vi "Pockels-Determine number of insertions for ref frame AO seq.vi"(7 "Prevent small final chunks (T)":bool, 9 "Nominal chunk length (points)":i32, 11 "Number of points in the original pockels modulation sequence":i32) -> (2 "Number of insertions":i32, 3 "Size of last chunk as % of nominal chunk size":dbl(slide) scale=0.0..100.0)   [LabVIEW 2020]
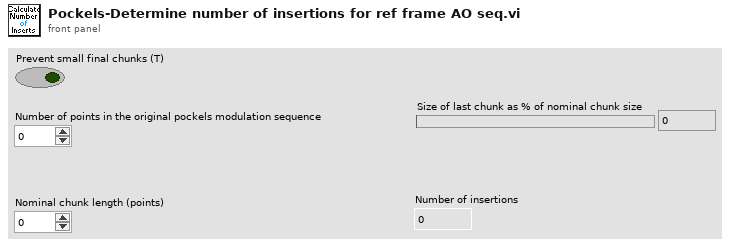
[diagram p1: front panel]
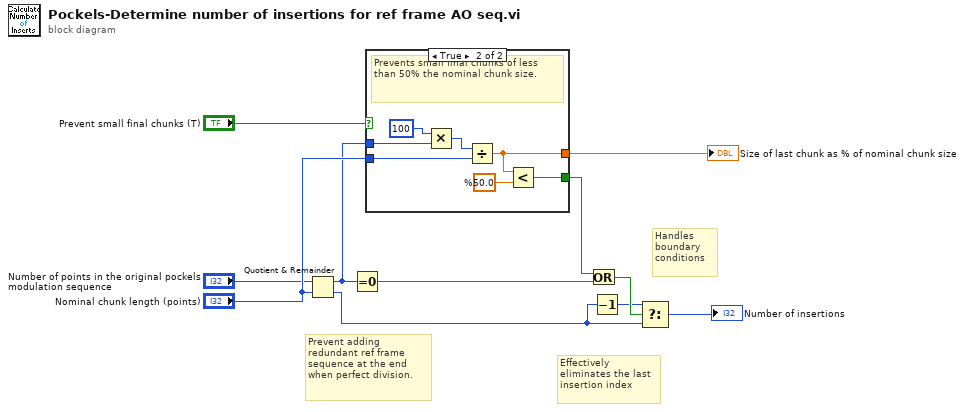
[diagram p0: block diagram]
diagram:
  # "Effectively eliminates the last insertion index"
  # "Prevent adding redundant ref frame sequence at the end when perfect division."
  # "Handles boundary conditions"
  n1 = Quotient & Remainder(x="Number of points in the original pockels modulation sequence", y="Nominal chunk length (points)") -> (x-y*floor(x/y)=w8:i32, floor(x/y)=w1:i32)
  n2 = Equal To 0?(x=w8) -> (x = 0?=w4:bool)
  n3 = case shown="True" "Prevent small final chunks (T)" {
    tunnel: [_ w17] -> w10
    tunnel: "Nominal chunk length (points)" -> [_ w16]
    tunnel: w8 -> [_ w15]
    tunnel: [_ w12] -> w3
    frame False {
    }
    frame True {
      w18 = 50.0  # %
      # "Prevents small final chunks of less than 50% the nominal chunk size."
      n4 = Multiply(x=100, y=w15) -> (x*y=w14:i32)
      n5 = Divide(x=w14, y=w16) -> (x/y=w17:dbl)
      n6 = Less?(x=w17, y=w18) -> (x < y?=w12:bool)
    }
  }
  "Size of last chunk as % of nominal chunk size" <- w10
  n7 = Or(x=w3, y=w4) -> (x .or. y?=w11:bool)
  n8 = Decrement(x=w1) -> (x-1=w7:i32)
  n9 = Select(t=w7, s=w11, f=w1) -> (s? t:f=→"Number of insertions":i32)
